vi "C - F temp conversion Sub VI.vi"() -> ()   [LabVIEW 2018]
panel:
  in  "stop":bool
  out "Temp C":dbl
  out "Temp F":dbl
  out "Temp C":dbl(slide) scale=0.0..200.0
  in  "Temp F":dbl(slide) scale=0.0..200.0
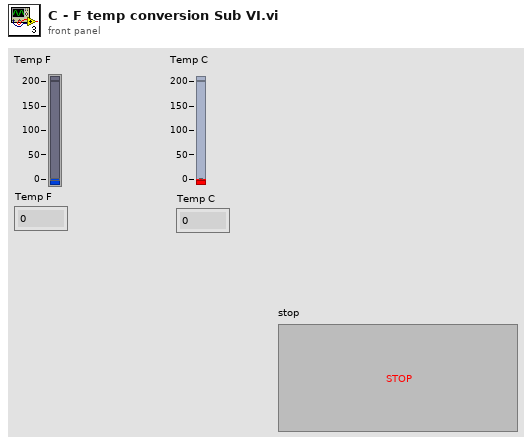
[diagram p1: front panel]
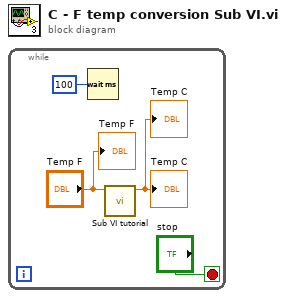
[diagram p0: block diagram]
diagram:
  n1 = while {
    stop <- "stop" stop-if-true
    n2 = Wait (ms)(milliseconds to wait=100) -> ()  [unwired: 1 out]
    n3 = call "Sub VI tutorial.vi"("Temp F"="Temp F") -> ("Temp C"=→"Temp C" →"Temp C":dbl)  [unwired: 10 in]
    "Temp F" <- "Temp F"
  }
